vi "Sample.vi"() -> ()   [LabVIEW 2020, in "CBOR.lvlib"]
doc: "CBOR Test"
uses:
  CBOR.lvlib
panel:
  out "# Bytes":i32
  out "# Bytes":i32
  out "JSON Data 2":string
  out "CBOR Data":string
  out "JSON Data":string
  in  "LV Data":T1={"Serial"={"Port"="COM3", "Baud Rate"=9800}, "TCP/IP"={"IP Address"="192.168.1.2", "Port"=8000}}
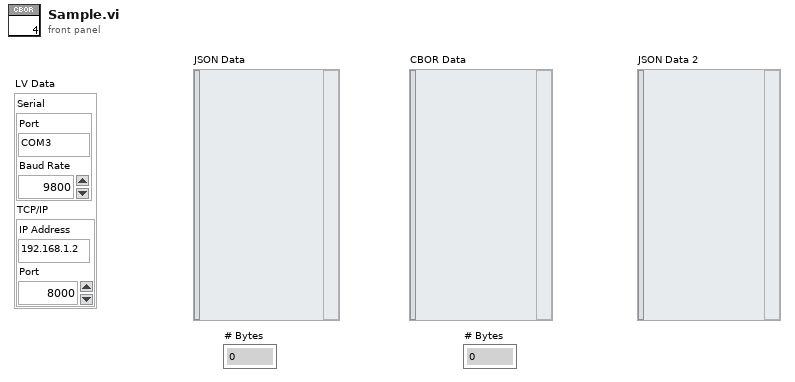
[diagram p1: front panel]
types:
  T1 = cluster{"Serial":cluster{"Port":string, "Baud Rate":i32}, "TCP/IP":cluster{"IP Address":string, "Port":i32}}
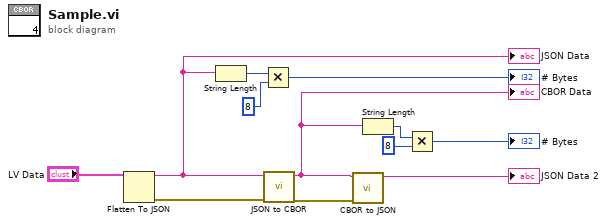
[diagram p0: block diagram]
diagram:
  n1 = Flatten To JSON(anything="LV Data") -> (JSON string=w8:string, 11:w11:errorcluster)  [unwired: 2 in]
  "JSON Data" <- w8
  n2 = String Length(string=w8) -> (length=w7:i32)
  n3 = Multiply(x=w7, y=8) -> (x*y=→"# Bytes":i32)
  n4 = call "JSON to CBOR.vi"("error in (no error)"=w11, "JSON Object"=w8) -> ("error out"=w10:errorcluster, "CBOR Hex"=w4:string)  [unwired: 8 in]
  "CBOR Data" <- w4
  n5 = call "CBOR to JSON.vi"("error in (no error)"=w10, "CBOR Hex"=w4) -> ("JSON Object"=→"JSON Data 2":string)  [unwired: 9 in]
  n6 = String Length(string=w4) -> (length=w3:i32)
  n7 = Multiply(x=w3, y=8) -> (x*y=→"# Bytes":i32)
